vi "Initialize.vi"(8 "error in (no error)":errorcluster, 11 "Relay-Box in":refnum<class "Relay-Box.lvclass">) -> (0 "error out":errorcluster, 3 "Relay-Box out":refnum<class "Relay-Box.lvclass">)   [LabVIEW 2019, in "Relay-Box.lvclass"]
uses:
  Relay-Box.lvclass
  <userlib>/LevyLab/D2XX-LV/D2XX-lv.lvlib
  <userlib>/LevyLab/D2XX-LV/private/Open Device (serial number).vi
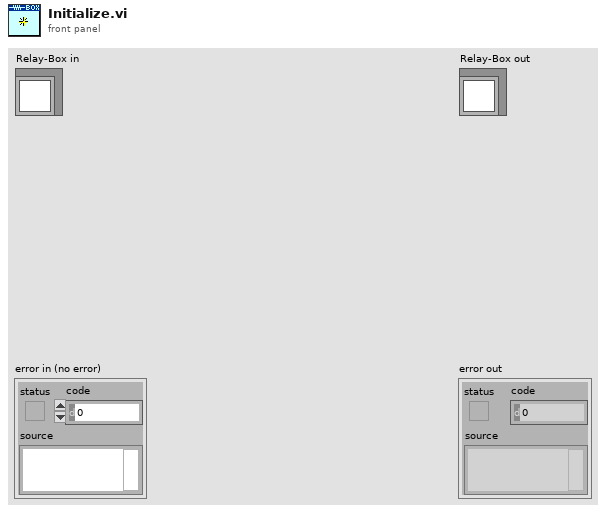
[diagram p1: front panel]
types:
  T1 = typedef "D2XX-lv.lvlib/Device Info.ctl" = cluster{"Serial Number":string, "COM port":string, "Description":string}
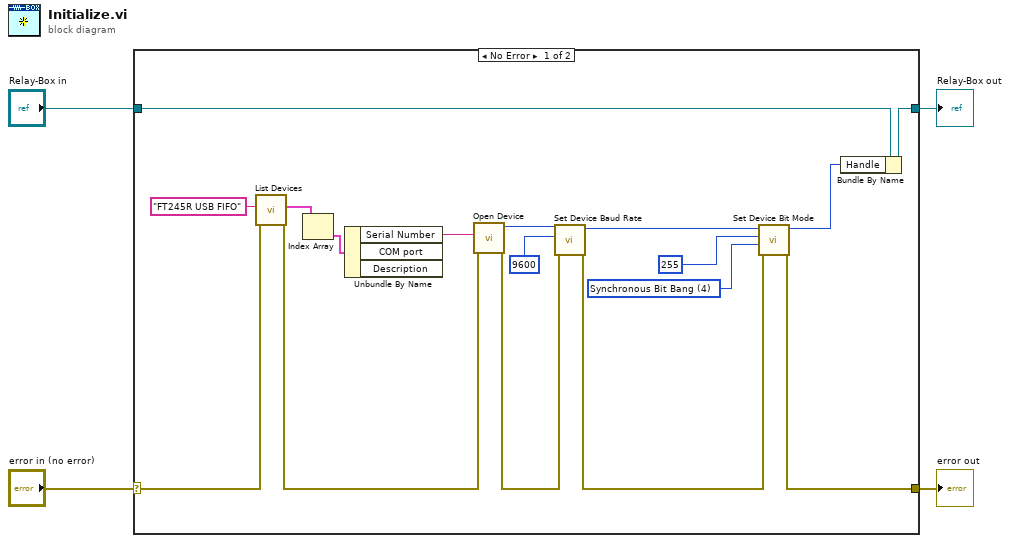
[diagram p0: block diagram]
diagram:
  n1 = case shown="No Error" "error in (no error)" {
    selector: "error in (no error)" -> [w6 w23]
    tunnel: [w8 w23] -> w3
    tunnel: [w21 w22] -> w1
    tunnel: "Relay-Box in" -> [w20 w22]
    frame No Error {
      w11 = u8 4 items=["Reset Bit Mode"=0, "Asynchronous Bit Bang"=1, "MPSSE"=2, "Synchronous Bit Bang"=4, "MCU Host Bus Emulation"=8, "Fast Opto-Isolated Serial"=16, "CBUS Bit Bang"=32, "Single Channel 245 Synchronous FIFO"=64] ("Bit Mode")
      n2 = call <userlib>:"List Devices.vi"("error in (no error)"=w6, "Filter (Device Description)"="FT245R USB FIFO") -> ("error out"=w18:errorcluster, "Devices"=w17:T1[])  [unwired: 8 in]
      n3 = Index Array(array=w17) -> (element=w16:T1)  [unwired: 1 in]
      n4 = Unbundle By Name(w16) -> ("Serial Number"=w15:string)  [unwired: 2 out]
      n5 = call-poly <userlib>:"Open Device.vi"("error in (no error)"=w18, "Device Serial Number"=w15) -> ("error out"=w12:errorcluster, "Handle"=w14:u32)  [unwired: 8 in]
      n6 = call <userlib>:"Set Device Baud Rate.vi"("error in (no error)"=w12, "Baud Rate"=u32 9600, "Handle"=w14) -> ("error out"=w9:errorcluster, "Handle out"=w10:u32)  [unwired: 7 in]
      n7 = call <userlib>:"Set Device Bit Mode.vi"("error in (no error)"=w9, "Bit Mode"=w11, "Bit Mode Mask"=u8 255, "Handle"=w10) -> ("error out"=w8:errorcluster, "Handle out"=w7:u32)  [unwired: 6 in]
      n8 = Bundle By Name(cluster=w20, "Handle"=w7) -> (w21:refnum<class "Relay-Box.lvclass">)
    }
    frame Error {
    }
  }
  "error out" <- w3
  "Relay-Box out" <- w1
